vi "Reboot.vi"() -> ()   [LabVIEW 2011]
doc: "ID=0x6008"
panel:
  out "label1":string="CAN中继状态"
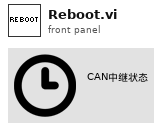
[diagram p1: front panel]
types:
  T1 = enum32{"Invalid", "Standard", "Closed", "Hidden", "Minimized", "Maximized"}
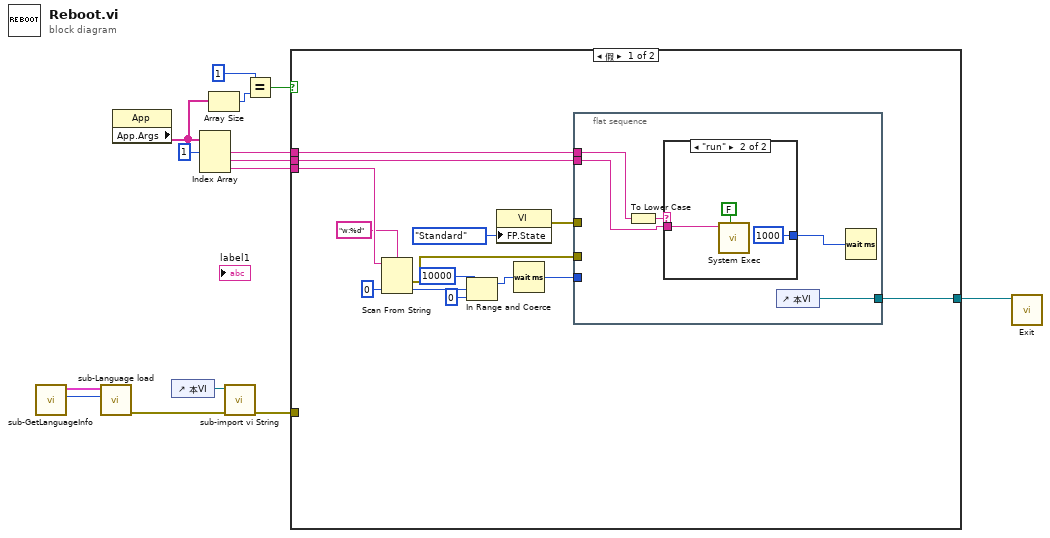
[diagram p0: block diagram]
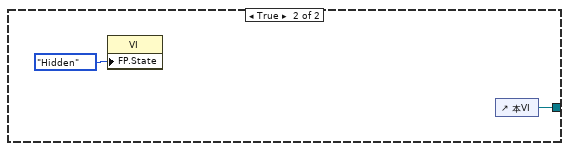
[diagram p3: hidden frame]
diagram:
  n1 = call "sub-GetLanguageInfo.vi"() -> ("selected"=w3:i32, "languages"=w2:cluster{string, "appended path":path, string}[])  [unwired: 10 in]
  n2 = call "sub-Language load.vi"("selected"=w3, "languages"=w2) -> ("error out"=w1:errorcluster)  [unwired: 9 in]
  n3 = property class="App"() -> ("App.Args"=w9:string[])  [unwired: 2 in, 2 out]
  n4 = control-ref of="本VI"() -> (w5:refnum<vi>)
  n5 = Index Array(array=w9, index #1=1 ("索引")) -> (element #1=w12:string, element #2=w11:string, element #3=w10:string)  [unwired: 2 in]
  n6 = Array Size(array=w9) -> (size(s)=w8:i32)
  n7 = call "sub-import vi String.vi"("error in (no error)"=w1, "vi ref"=w5) -> ("error out"=w4:errorcluster)  [unwired: 9 in]
  n8 = Equal?(x=1, y=w8) -> (x = y?=w6:bool)
  n9 = case shown="假" w6 {
    tunnel: [w28 w38] -> w14
    tunnel: w12 -> [w24 _]
    tunnel: w11 -> [w23 _]
    tunnel: w10 -> [w22 _]
    tunnel: w4 -> [_ _]
    frame False {
      n10 = Scan From String(format string="w:%d" ("格式字符串"), input string=w22, default 1=u32 0 ("等待时间（毫秒）")) -> (error out=w16:errorcluster, output 1=w20:u32)  [unwired: 2 in, 2 out]
      n11 = In Range and Coerce(upper limit=u32 10000 ("上限"), x=w20, lower limit=u32 0 ("下限")) -> (coerced(x)=w17:u32)  [unwired: 1 out]
      n12 = property class="VI"("FP.State"=T1."Standard" ("前面板窗口:状态")) -> (error out=w26:errorcluster)  [unwired: 2 in, 1 out]
      n13 = Wait (ms)(milliseconds to wait=w17) -> (millisecond timer value=w25:u32)
      n14 = flat-sequence {
        tunnel: [w33] -> w28
        tunnel: w26 -> [_]
        tunnel: w25 -> [_]
        tunnel: w24 -> [w31]
        tunnel: w23 -> [w30]
        tunnel: w16 -> [_]
        frame #0 {
          n15 = To Lower Case(string=w31) -> (all lower case string=w32:string)
          n16 = case shown="\"run\"" w32 {
            tunnel: w30 -> [_ w36]
            tunnel: [_ u32 1000 ("等待时间（毫秒）")] -> w29
            frame "假", Default {
            }
            frame "run" {
              n17 = call <vilib>:"System Exec.vi"("wait until completion? (T)"=FALSE, "command line"=w36) -> ()  [unwired: 6 in, 4 out]
            }
          }
          n18 = control-ref of="本VI"() -> (w33:refnum<vi>)
          n19 = Wait (ms)(milliseconds to wait=w29) -> ()  [unwired: 1 out]
        }
      }
    }
    frame True {
      n20 = property class="VI"("FP.State"=T1."Hidden" ("前面板窗口:状态")) -> ()  [unwired: 2 in, 2 out]
      n21 = control-ref of="本VI"() -> (w38:refnum<vi>)
    }
  }
  n22 = call "Exit.vi"("VI引用"=w14) -> ()  [unwired: 10 in, 1 out]
